vi "Exam.vi"() -> ()   [LabVIEW 2019]
panel:
  out "Timer4":u8
  out "Timer3":u8
  out "Timer2":u8
  out "Timer1":u8
  out "Signal1 4":cluster{"Red":bool, "Amber":bool, "Green":bool}
  out "Signal1 3":cluster{"Red":bool, "Amber":bool, "Green":bool}
  out "Signal1 2":cluster{"Red":bool, "Amber":bool, "Green":bool}
  out "Signal1":cluster{"Red":bool, "Amber":bool, "Green":bool}
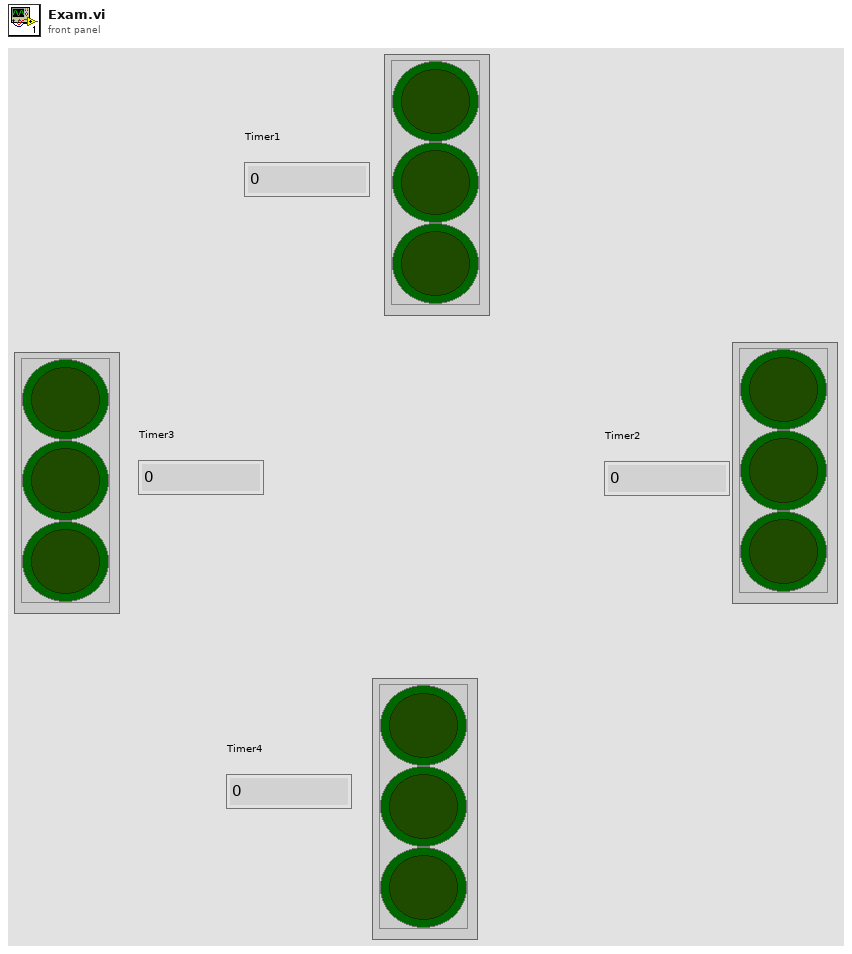
[diagram p1: front panel]
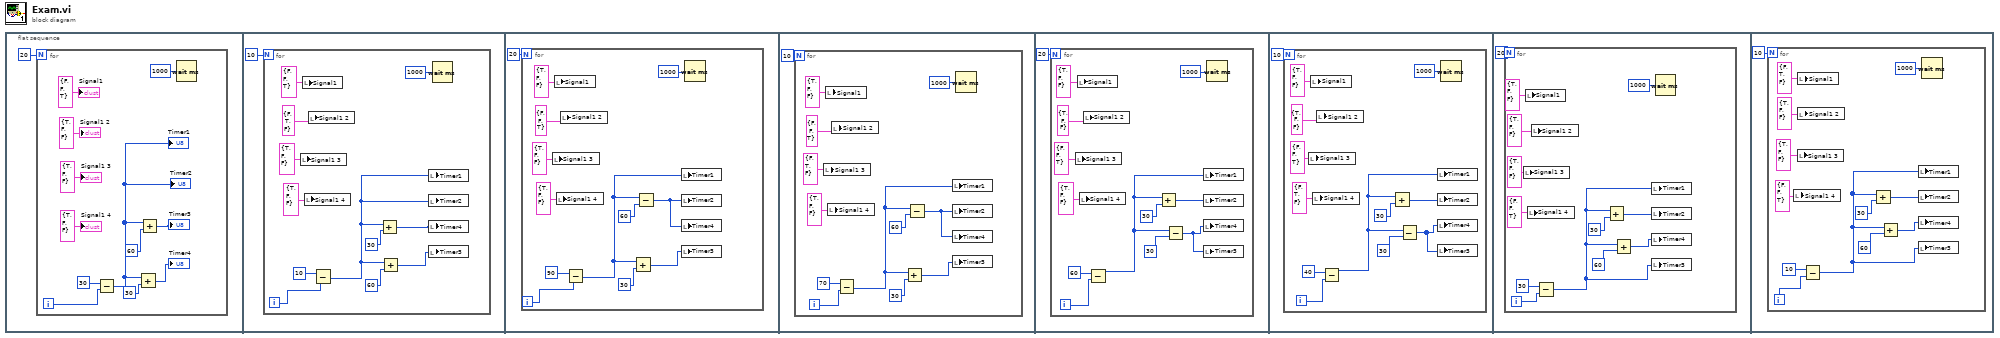
[diagram p0: block diagram]
diagram:
  n1 = flat-sequence {
    frame #0 {
      n2 = for {
        N: 20 -> [_]
        i -> [w5]
        n3 = Subtract(x=30, y=w5) -> (x-y=w7:i32)
        "Timer1" <- w7
        "Timer2" <- w7
        n4 = Add(x=w7, y=30) -> (x+y=→"Timer4":i32)
        n5 = Add(x=w7, y=60) -> (x+y=→"Timer3":i32)
        n6 = Wait (ms)(milliseconds to wait=u32 1000) -> ()  [unwired: 1 out]
        "Signal1" <- cluster{"Red":bool, "Amber":bool, "Green":bool} {"Red"=FALSE, "Amber"=FALSE, "Green"=TRUE} ("Signal1")
        "Signal1 2" <- cluster{"Red":bool, "Amber":bool, "Green":bool} {"Red"=TRUE, "Amber"=FALSE, "Green"=FALSE} ("Signal1 2")
        "Signal1 3" <- cluster{"Red":bool, "Amber":bool, "Green":bool} {"Red"=TRUE, "Amber"=FALSE, "Green"=FALSE} ("Signal1 3")
        "Signal1 4" <- cluster{"Red":bool, "Amber":bool, "Green":bool} {"Red"=TRUE, "Amber"=FALSE, "Green"=FALSE} ("Signal1 4")
      }
    }
    frame #1 {
      n7 = for {
        N: 10 -> [_]
        i -> [w21]
        n8 = local write "Signal1 3"(cluster{"Red":bool, "Amber":bool, "Green":bool} {"Red"=TRUE, "Amber"=FALSE, "Green"=FALSE} ("Signal1 3")) -> ()
        n9 = local write "Signal1"(cluster{"Red":bool, "Amber":bool, "Green":bool} {"Red"=FALSE, "Amber"=FALSE, "Green"=TRUE} ("Signal1")) -> ()
        n10 = local write "Signal1 4"(cluster{"Red":bool, "Amber":bool, "Green":bool} {"Red"=TRUE, "Amber"=FALSE, "Green"=FALSE} ("Signal1 4")) -> ()
        n11 = local write "Signal1 2"(cluster{"Red":bool, "Amber":bool, "Green":bool} {"Red"=FALSE, "Amber"=TRUE, "Green"=FALSE} ("Signal1 3")) -> ()
        n12 = Subtract(x=10, y=w21) -> (x-y=w17:i32)
        n13 = Add(x=w17, y=30) -> (x+y=w19:i32)
        n14 = Add(x=w17, y=60) -> (x+y=w18:i32)
        n15 = local write "Timer1"(w17) -> ()
        n16 = local write "Timer2"(w17) -> ()
        n17 = local write "Timer4"(w19) -> ()
        n18 = local write "Timer3"(w18) -> ()
        n19 = Wait (ms)(milliseconds to wait=u32 1000) -> ()  [unwired: 1 out]
      }
    }
    frame #2 {
      n20 = for {
        N: 20 -> [_]
        i -> [w34]
        n21 = local write "Signal1 3"(cluster{"Red":bool, "Amber":bool, "Green":bool} {"Red"=TRUE, "Amber"=FALSE, "Green"=FALSE} ("Signal1 3")) -> ()
        n22 = local write "Signal1"(cluster{"Red":bool, "Amber":bool, "Green":bool} {"Red"=TRUE, "Amber"=FALSE, "Green"=FALSE} ("Signal1")) -> ()
        n23 = local write "Signal1 4"(cluster{"Red":bool, "Amber":bool, "Green":bool} {"Red"=TRUE, "Amber"=FALSE, "Green"=FALSE} ("Signal1 4")) -> ()
        n24 = local write "Signal1 2"(cluster{"Red":bool, "Amber":bool, "Green":bool} {"Red"=FALSE, "Amber"=FALSE, "Green"=TRUE} ("Signal1 3")) -> ()
        n25 = Subtract(x=90, y=w34) -> (x-y=w30:i32)
        n26 = Add(x=w30, y=30) -> (x+y=w32:i32)
        n27 = Subtract(x=w30, y=60) -> (x-y=w28:i32)
        n28 = local write "Timer1"(w30) -> ()
        n29 = local write "Timer2"(w28) -> ()
        n30 = local write "Timer4"(w28) -> ()
        n31 = local write "Timer3"(w32) -> ()
        n32 = Wait (ms)(milliseconds to wait=u32 1000) -> ()  [unwired: 1 out]
      }
    }
    frame #3 {
      n33 = for {
        N: 10 -> [_]
        i -> [w41]
        n34 = local write "Signal1 3"(cluster{"Red":bool, "Amber":bool, "Green":bool} {"Red"=FALSE, "Amber"=TRUE, "Green"=FALSE} ("Signal1 3")) -> ()
        n35 = local write "Signal1"(cluster{"Red":bool, "Amber":bool, "Green":bool} {"Red"=TRUE, "Amber"=FALSE, "Green"=FALSE} ("Signal1")) -> ()
        n36 = local write "Signal1 4"(cluster{"Red":bool, "Amber":bool, "Green":bool} {"Red"=TRUE, "Amber"=FALSE, "Green"=FALSE} ("Signal1 4")) -> ()
        n37 = local write "Signal1 2"(cluster{"Red":bool, "Amber":bool, "Green":bool} {"Red"=FALSE, "Amber"=FALSE, "Green"=TRUE} ("Signal1 3")) -> ()
        n38 = Subtract(x=70, y=w41) -> (x-y=w50:i32)
        n39 = Add(x=w50, y=30) -> (x+y=w48:i32)
        n40 = Subtract(x=w50, y=60) -> (x-y=w52:i32)
        n41 = local write "Timer1"(w50) -> ()
        n42 = local write "Timer2"(w52) -> ()
        n43 = local write "Timer4"(w52) -> ()
        n44 = local write "Timer3"(w48) -> ()
        n45 = Wait (ms)(milliseconds to wait=u32 1000) -> ()  [unwired: 1 out]
      }
    }
    frame #4 {
      n46 = for {
        N: 20 -> [_]
        i -> [w55]
        n47 = local write "Signal1 3"(cluster{"Red":bool, "Amber":bool, "Green":bool} {"Red"=FALSE, "Amber"=FALSE, "Green"=TRUE} ("Signal1 3")) -> ()
        n48 = local write "Signal1"(cluster{"Red":bool, "Amber":bool, "Green":bool} {"Red"=TRUE, "Amber"=FALSE, "Green"=FALSE} ("Signal1")) -> ()
        n49 = local write "Signal1 4"(cluster{"Red":bool, "Amber":bool, "Green":bool} {"Red"=TRUE, "Amber"=FALSE, "Green"=FALSE} ("Signal1 4")) -> ()
        n50 = local write "Signal1 2"(cluster{"Red":bool, "Amber":bool, "Green":bool} {"Red"=TRUE, "Amber"=FALSE, "Green"=FALSE} ("Signal1 3")) -> ()
        n51 = Subtract(x=60, y=w55) -> (x-y=w58:i32)
        n52 = Add(x=w58, y=30) -> (x+y=w56:i32)
        n53 = Subtract(x=w58, y=30) -> (x-y=w54:i32)
        n54 = local write "Timer1"(w58) -> ()
        n55 = local write "Timer2"(w56) -> ()
        n56 = local write "Timer4"(w54) -> ()
        n57 = local write "Timer3"(w54) -> ()
        n58 = Wait (ms)(milliseconds to wait=u32 1000) -> ()  [unwired: 1 out]
      }
    }
    frame #5 {
      n59 = for {
        N: 10 -> [_]
        i -> [w67]
        n60 = local write "Signal1 3"(cluster{"Red":bool, "Amber":bool, "Green":bool} {"Red"=FALSE, "Amber"=FALSE, "Green"=TRUE} ("Signal1 3")) -> ()
        n61 = local write "Signal1"(cluster{"Red":bool, "Amber":bool, "Green":bool} {"Red"=TRUE, "Amber"=FALSE, "Green"=FALSE} ("Signal1")) -> ()
        n62 = local write "Signal1 4"(cluster{"Red":bool, "Amber":bool, "Green":bool} {"Red"=FALSE, "Amber"=TRUE, "Green"=FALSE} ("Signal1 4")) -> ()
        n63 = local write "Signal1 2"(cluster{"Red":bool, "Amber":bool, "Green":bool} {"Red"=TRUE, "Amber"=FALSE, "Green"=FALSE} ("Signal1 3")) -> ()
        n64 = Subtract(x=40, y=w67) -> (x-y=w75:i32)
        n65 = Add(x=w75, y=30) -> (x+y=w77:i32)
        n66 = Subtract(x=w75, y=30) -> (x-y=w78:i32)
        n67 = local write "Timer1"(w75) -> ()
        n68 = local write "Timer2"(w77) -> ()
        n69 = local write "Timer4"(w78) -> ()
        n70 = local write "Timer3"(w78) -> ()
        n71 = Wait (ms)(milliseconds to wait=u32 1000) -> ()  [unwired: 1 out]
      }
    }
    frame #6 {
      n72 = for {
        N: 20 -> [_]
        i -> [w84]
        n73 = local write "Signal1 3"(cluster{"Red":bool, "Amber":bool, "Green":bool} {"Red"=TRUE, "Amber"=FALSE, "Green"=FALSE} ("Signal1 3")) -> ()
        n74 = local write "Signal1"(cluster{"Red":bool, "Amber":bool, "Green":bool} {"Red"=TRUE, "Amber"=FALSE, "Green"=FALSE} ("Signal1")) -> ()
        n75 = local write "Signal1 4"(cluster{"Red":bool, "Amber":bool, "Green":bool} {"Red"=FALSE, "Amber"=FALSE, "Green"=TRUE} ("Signal1 4")) -> ()
        n76 = local write "Signal1 2"(cluster{"Red":bool, "Amber":bool, "Green":bool} {"Red"=TRUE, "Amber"=FALSE, "Green"=FALSE} ("Signal1 2")) -> ()
        n77 = Subtract(x=30, y=w84) -> (x-y=w80:i32)
        n78 = Add(x=w80, y=30) -> (x+y=w86:i32)
        n79 = Add(x=w80, y=60) -> (x+y=w85:i32)
        n80 = local write "Timer1"(w80) -> ()
        n81 = local write "Timer2"(w86) -> ()
        n82 = local write "Timer4"(w85) -> ()
        n83 = local write "Timer3"(w80) -> ()
        n84 = Wait (ms)(milliseconds to wait=u32 1000) -> ()  [unwired: 1 out]
      }
    }
    frame #7 {
      n85 = for {
        N: 10 -> [_]
        i -> [w93]
        n86 = local write "Signal1 4"(cluster{"Red":bool, "Amber":bool, "Green":bool} {"Red"=FALSE, "Amber"=FALSE, "Green"=TRUE} ("Signal1 4")) -> ()
        n87 = local write "Signal1 3"(cluster{"Red":bool, "Amber":bool, "Green":bool} {"Red"=TRUE, "Amber"=FALSE, "Green"=FALSE} ("Signal1 3")) -> ()
        n88 = local write "Signal1"(cluster{"Red":bool, "Amber":bool, "Green":bool} {"Red"=FALSE, "Amber"=TRUE, "Green"=FALSE} ("Signal1")) -> ()
        n89 = local write "Signal1 2"(cluster{"Red":bool, "Amber":bool, "Green":bool} {"Red"=TRUE, "Amber"=FALSE, "Green"=FALSE} ("Signal1 2")) -> ()
        n90 = Subtract(x=10, y=w93) -> (x-y=w104:i32)
        n91 = Add(x=w104, y=30) -> (x+y=w102:i32)
        n92 = Add(x=w104, y=60) -> (x+y=w103:i32)
        n93 = local write "Timer1"(w104) -> ()
        n94 = local write "Timer2"(w102) -> ()
        n95 = local write "Timer4"(w103) -> ()
        n96 = local write "Timer3"(w104) -> ()
        n97 = Wait (ms)(milliseconds to wait=u32 1000) -> ()  [unwired: 1 out]
      }
    }
  }
